vi "CLAD Exercise 3-6.vi"() -> ()   [LabVIEW 2014]
panel:
  in  "stop":bool
  in  "Enum":T1(ring)
  out "Converted Temperature":dbl
  in  "Initial Temperature":dbl
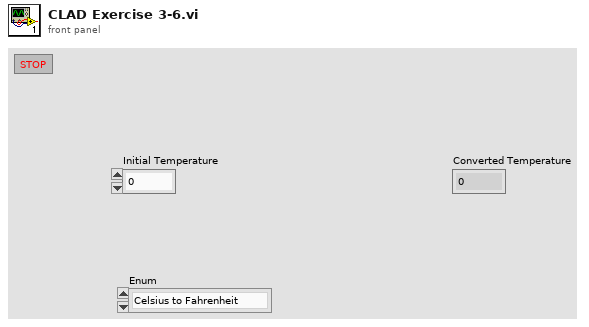
[diagram p1: front panel]
types:
  T1 = enum16{"Celsius to Fahrenheit", "Fahrenheit to Celsius", "Fahrenheit to Kelvin", "Celsius to Kelvin"}
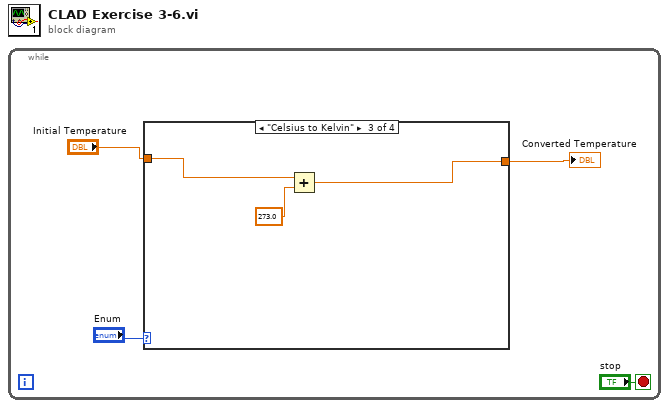
[diagram p0: block diagram]
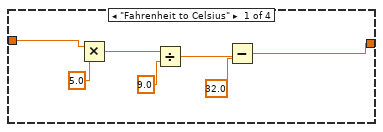
[diagram p2: hidden frame]
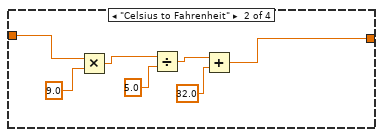
[diagram p3: hidden frame]
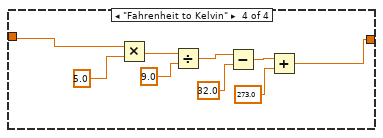
[diagram p4: hidden frame]
diagram:
  n1 = while {
    stop <- "stop" stop-if-true
    n2 = case shown="\"Celsius to Kelvin\"" "Enum" {
      tunnel: "Initial Temperature" -> [w6 w15 w20 w23]
      tunnel: [w5 w12 w19 w22] -> w3
      frame "Fahrenheit to Celsius" {
        n3 = Multiply(x=w6, y=5.0) -> (x*y=w9:dbl)
        n4 = Divide(x=w9, y=9.0) -> (x/y=w7:dbl)
        n5 = Subtract(x=w7, y=32.0) -> (x-y=w5:dbl)
      }
      frame "Celsius to Fahrenheit" {
        n6 = Multiply(x=w15, y=9.0) -> (x*y=w17:dbl)
        n7 = Divide(x=w17, y=5.0) -> (x/y=w14:dbl)
        n8 = Add(x=w14, y=32.0) -> (x+y=w12:dbl)
      }
      frame "Celsius to Kelvin" {
        n9 = Add(x=w20, y=273.0) -> (x+y=w19:dbl)
      }
      frame "Fahrenheit to Kelvin" {
        n10 = Multiply(x=w23, y=5.0) -> (x*y=w26:dbl)
        n11 = Divide(x=w26, y=9.0) -> (x/y=w27:dbl)
        n12 = Subtract(x=w27, y=32.0) -> (x-y=w29:dbl)
        n13 = Add(x=w29, y=273.0) -> (x+y=w22:dbl)
      }
    }
    "Converted Temperature" <- w3
  }
